vi "IntakeExecuteLogic.vi"(9 "HaveAlgaeSensor":bool, 11 "HaveCoralSensor":bool) -> (1 "MotorDemandRight":dbl, 2 "MotorDemandLeft":dbl, 3 "MotorDemandTop":dbl, 4 "CurrentState":T1)   [LabVIEW 2023]
doc: "Intake Commands go in and Motor Demands are outputted\nOutputs:\n--MotorDemandTop--numeric\n--MotorDemandLeft--numeric\nMotorDemandRight--numeric"
uses:
  <vilib>/Rock Robotics/WPI/ThirdParty/JAS_Junk/TrajLib/Trajectory_Library.lvlib
  IntakeStates.ctl
  IntakeGlobal.vi
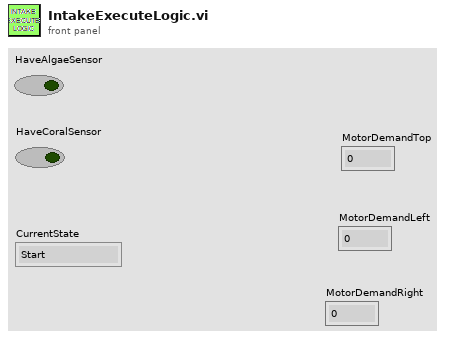
[diagram p1: front panel]
types:
  T1 = typedef "IntakeStates.ctl" = enum16{"Start", "WaitForCommand", "IntakeCoral", "IntakeAlgae", "WaitForCoral", "WaitForAlgae", "DepositCoral", "DepositAlgae", "DepositCoralTimer", "DepositAlgaeTimer"}
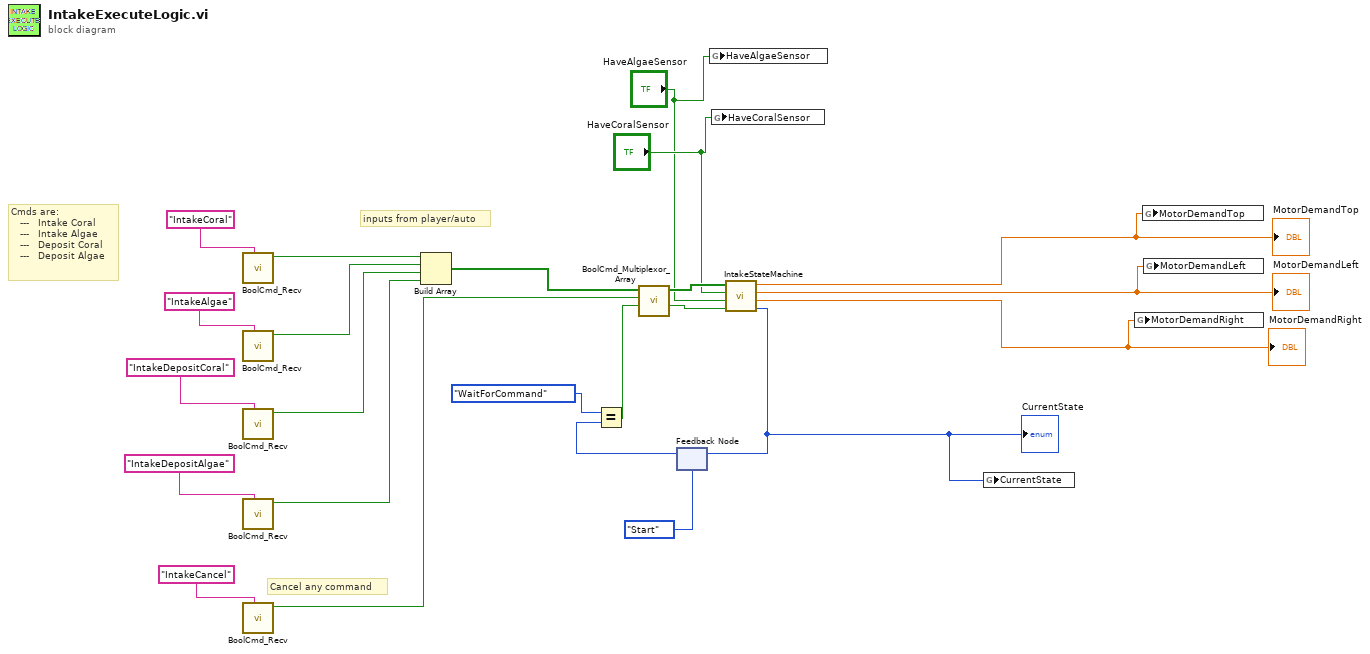
[diagram p0: block diagram]
diagram:
  # "Cmds are:\n   ---   Intake Coral\n   ---   Intake Algae\n   ---   Deposit Coral\n   ---   Deposit Algae"
  # "inputs from player/auto"
  # "Cancel any command"
  n1 = call <vilib>:"BoolCmd_Recv.vi"("Command Name"="IntakeCoral") -> ("New Request"=w5:bool)  [unwired: 9 in, 1 out]
  n2 = call <vilib>:"BoolCmd_Recv.vi"("Command Name"="IntakeAlgae") -> ("New Request"=w4:bool)  [unwired: 9 in, 1 out]
  n3 = call <vilib>:"BoolCmd_Recv.vi"("Command Name"="IntakeDepositCoral") -> ("New Request"=w3:bool)  [unwired: 9 in, 1 out]
  n4 = call <vilib>:"BoolCmd_Recv.vi"("Command Name"="IntakeDepositAlgae") -> ("New Request"=w2:bool)  [unwired: 9 in, 1 out]
  n5 = call <vilib>:"BoolCmd_Recv.vi"("Command Name"="IntakeCancel") -> ("New Request"=w1:bool)  [unwired: 9 in, 1 out]
  n6 = Build Array(w5, w4, w3, w2) -> (w20:bool[])
  n7 = feedback #1(IntakeStates."Start" ("CurrentState")) -> (w15:T1)
  n8 = Equal?(x=IntakeStates."WaitForCommand", y=w15) -> (x = y?=w13:bool)
  n9 = call <vilib>:"BoolCmd_Multiplexor_Array.vi"("Ready"=w13, "Command Cancel"=w1, "Commands"=w20) -> ("Do Cancel"=w17:bool, "Do Command"=w18:bool[])  [unwired: 7 in]
  n10 = global write "IntakeGlobal.vi" "HaveAlgaeSensor"("HaveAlgaeSensor") -> ()
  n11 = global write "IntakeGlobal.vi" "HaveCoralSensor"("HaveCoralSensor") -> ()
  n12 = call "IntakeStateMachine.vi"("IntakeCancel"=w17, "HaveAlgaeSensor"="HaveAlgaeSensor", "HaveCoralSensor"="HaveCoralSensor", "IntakeCommands"=w18) -> ("CurrentState"=w6:T1, "RightMotorDemand"=w9:dbl, "LeftMotorDemand"=w10:dbl, "TopMotorDemand"=w11:dbl)  [unwired: 4 in]
  "MotorDemandLeft" <- w10
  "MotorDemandRight" <- w9
  "CurrentState" <- w6
  "MotorDemandTop" <- w11
  n13 = feedback-in #1(w6) -> ()
  n14 = global write "IntakeGlobal.vi" "CurrentState"(w6) -> ()
  n15 = global write "IntakeGlobal.vi" "MotorDemandRight"(w9) -> ()
  n16 = global write "IntakeGlobal.vi" "MotorDemandTop"(w11) -> ()
  n17 = global write "IntakeGlobal.vi" "MotorDemandLeft"(w10) -> ()
